vi "acquire-sequence-to-disk-subvi.vi"(0 "Image Size":T4={"H Bin"=1.0, "V Bin"=1.0, "Left"=1.0, "Right"=1024.0, "Top"=1.0, "Bottom"=1024.0} {"V Bin" min=0.0; "H Bin" min=0.0 step=1.0}, 1 "Description Info":string, 2 "Operation":enum16{"Start", "Continue", "Finish"}(ring), 3 "Number of frames to acquire":i32, 5 "Display?":bool, 7 "State In":T1 {"Height" format="%.2f"; "Width" format="%.2f"}, 9 "Frames per acquisition file":u32, 11 "Sequence files handle":T5, 12 "Pressing stop \nautomatically runs finish?":bool=TRUE, 13 "Display Window Title":string="Acquired Image", 14 "Display Window Number":i32) -> (4 "Done?":bool, 6 "State Out":T1 {"Height" format="%.2f"; "Width" format="%.2f"}, 10 "Sequence files handle out":T5, 15 "Error Out":errorcluster)   [LabVIEW 2014]
uses:
  ctt's/Video acquisition state1.ctl
  <vilib>/vision/Image Controls.llb/IMAQ Image.ctl
  ctt's/Header2 file.ctl
  Globals/Initilize Globals.vi
  Stage Control/stage-controller-globals.vi
  Shutter Control/Shutter SubVIs/Global Shutter Variables - SubVI.vi
  Globals/flow-rate-global.vi
  Globals/Andor Camera Temperature.vi
  Globals/hardware names - global.vi
panel:
  in  "Laser Shutter (to get strings only)":T3(radio)
  out "Frame interval (ms)":i16
  out "TTB element zero":u32
  out "Time of 1st frame":dbl
  out "Frames Acquired":u32(slide) scale=0.0..10000.0
  in  "Stop":bool
  out "Sequence files directory path":path
  # "Outputs"
  # "Inputs"
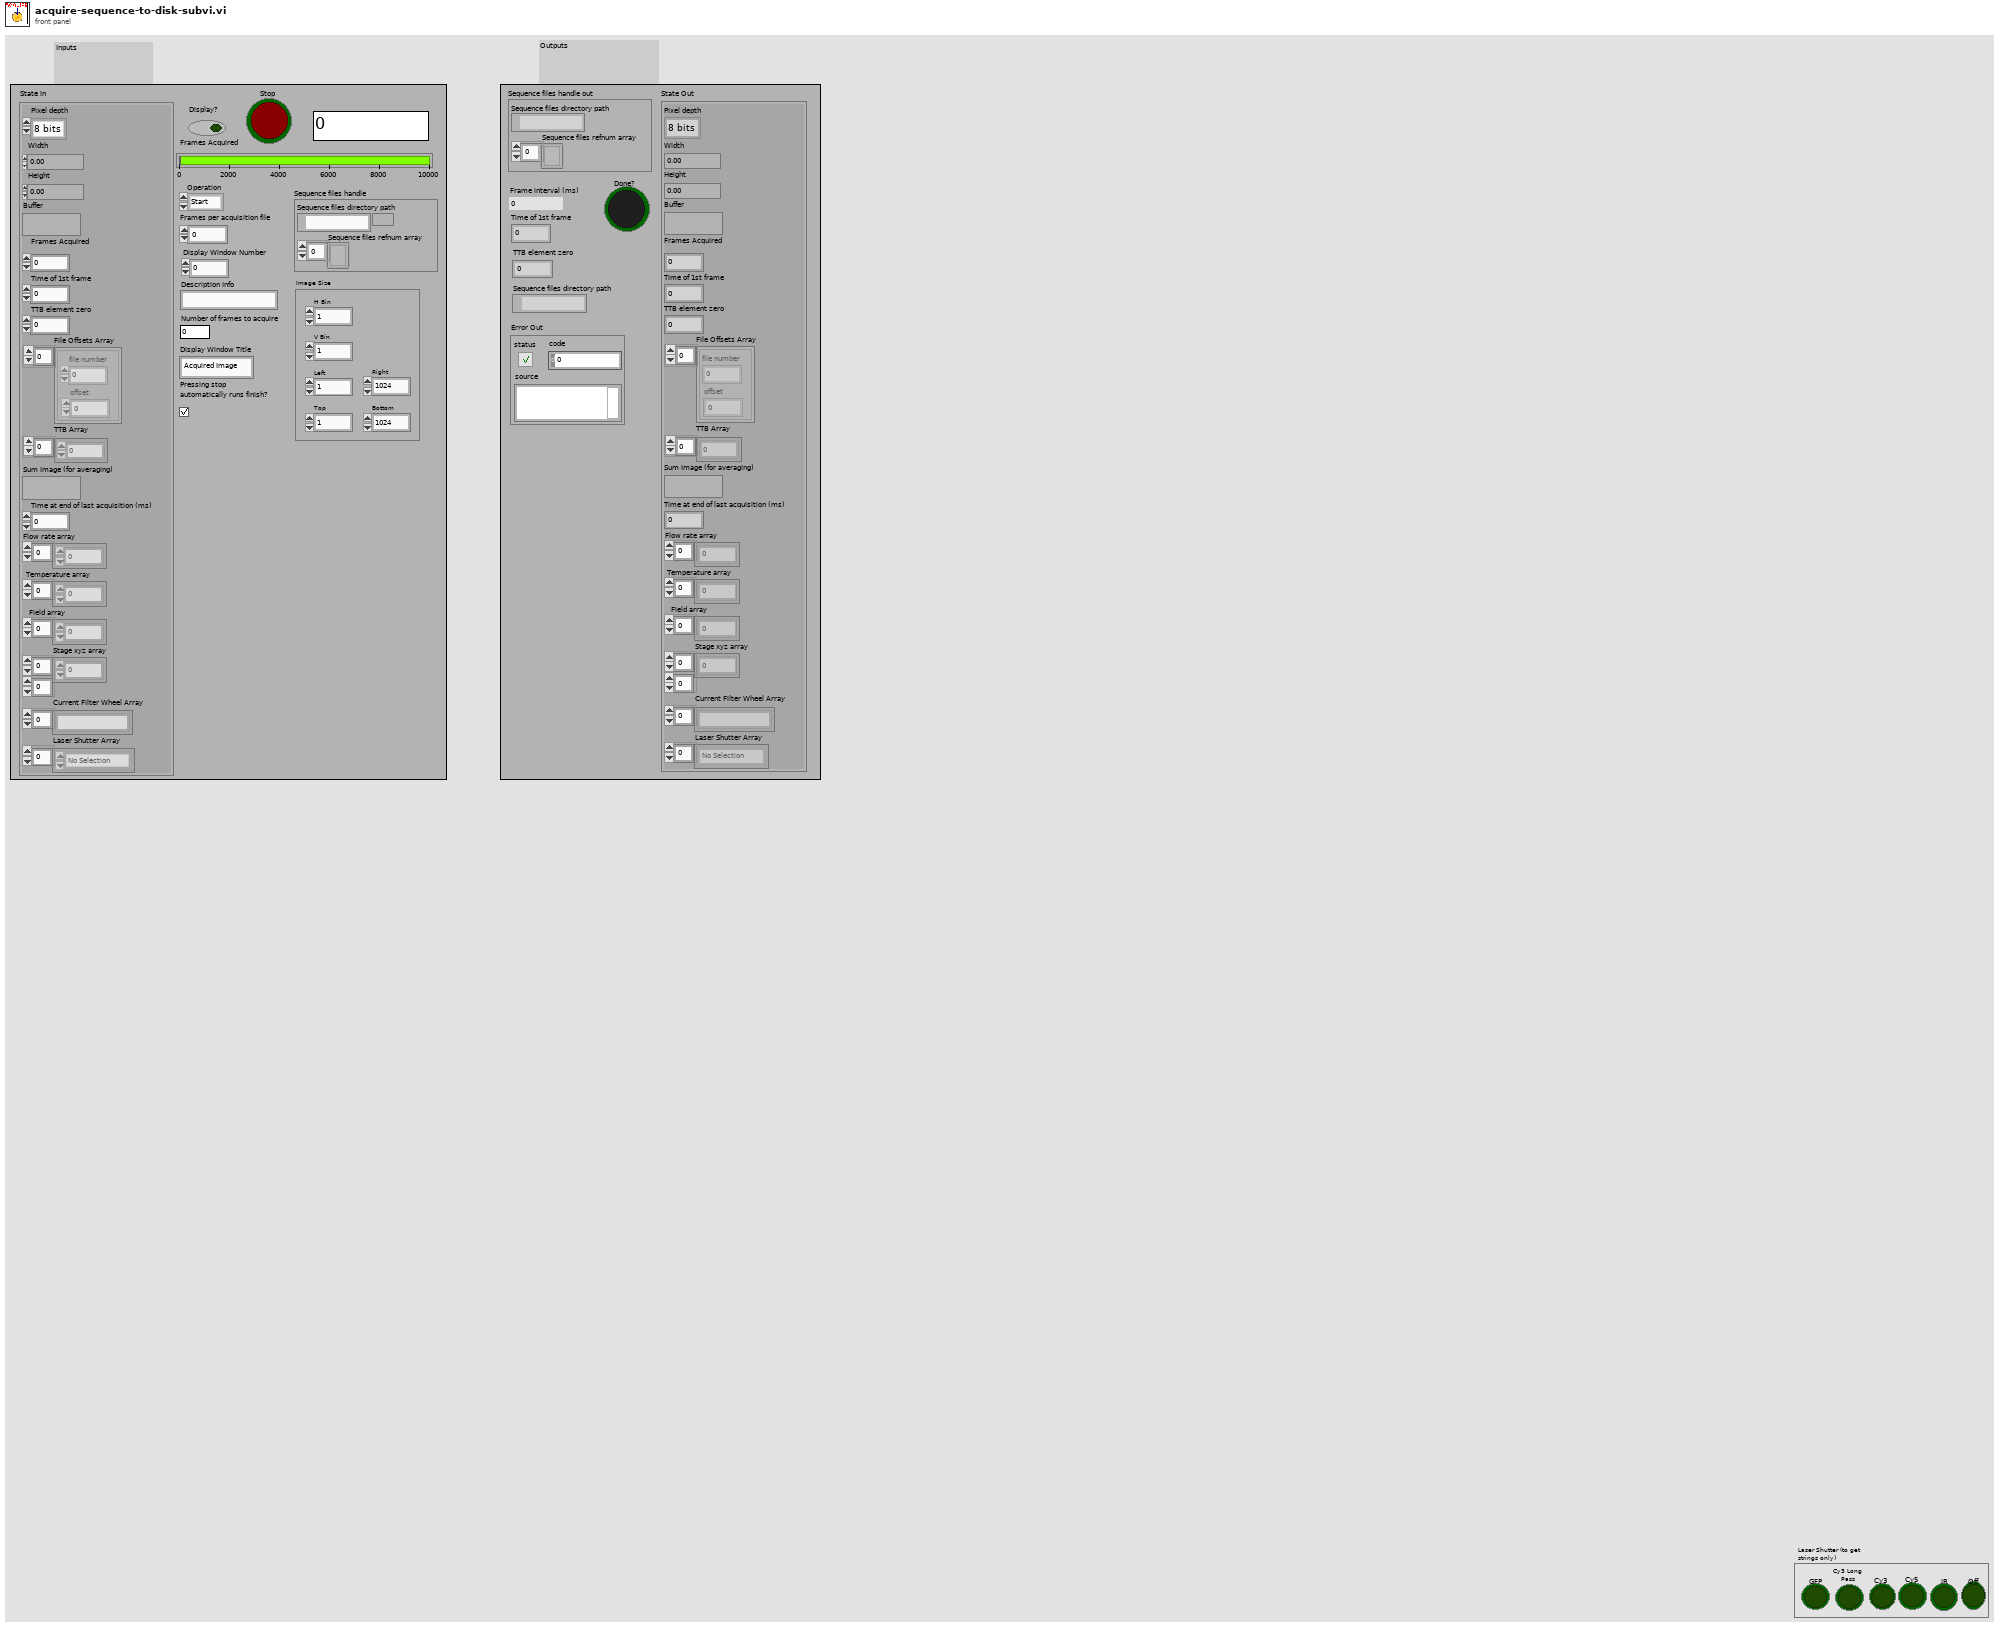
[diagram p1: front panel]
types:
  T1 = typedef "Video acquisition state1.ctl" = cluster{"Pixel depth":enum32{"8 bits", "16 bits", "Float", "Complex", "RGB Chunky", "Compressed"}, "Width":dbl, "Height":dbl, "Buffer":T2, "Frames Acquired":u32, "Time of 1st frame":dbl, "TTB element zero":u32, "File Offsets Array":cluster{"offset":i32, "file number":u8}[], "TTB Array":u32[], "Sum Image (for averaging)":T2, "Time at end of last acquisition (ms)":u32, "Flow rate array":dbl[], "Temperature array":dbl[], "Field array":u16[], "Stage xyz array":dbl[][], "Current Filter Wheel Array":string[], "Laser Shutter Array":enum32{"No Selection", "GFP", "Cy3 Long \nPass", "Cy3", "Cy5", "Off", "IR"}[]}
  T2 = typedef "IMAQ Image.ctl" = refnum<image>
  T3 = enum32{"No Selection", "GFP", "Cy3 Long \nPass", "Cy3", "Cy5", "Off", "IR"}
  T4 = cluster{"H Bin":dbl, "V Bin":dbl, "Left":dbl, "Right":dbl, "Top":dbl, "Bottom":dbl}
  T5 = cluster{"Sequence files directory path":path, "Sequence files refnum array":refnum<file>[]}
  T6 = enum32{"8 bits", "16 bits", "Float", "Complex", "RGB Chunky", "Compressed"}
  T7 = enum32{"No Selection", "GFP", "Cy3 Long \nPass", "Cy3", "Cy5", "Off", "IR"}[]
  T8 = typedef "laser shutters.ctl" = enum32{"No Selection", "GFP", "Cy3 Long \nPass", "Cy3", "Cy5", "Off", "IR"}
  T9 = typedef "Header2 file.ctl" = cluster{"Camera":string, "Microscope":string, "Microscope software version":string, "Flow rate array":dbl[], "Temperature array":dbl[], "Field array":u16[], "Is header2 info present?":bool, "Description Info":string, "Stage xyz array":dbl[][], "Current Filter Wheel Array":string[], "Laser Shutter Array":enum32{"No Selection", "GFP", "Cy3 Long \nPass", "Cy3", "Cy5", "Off", "IR"}[], "Laser Shutter Names":string[]}
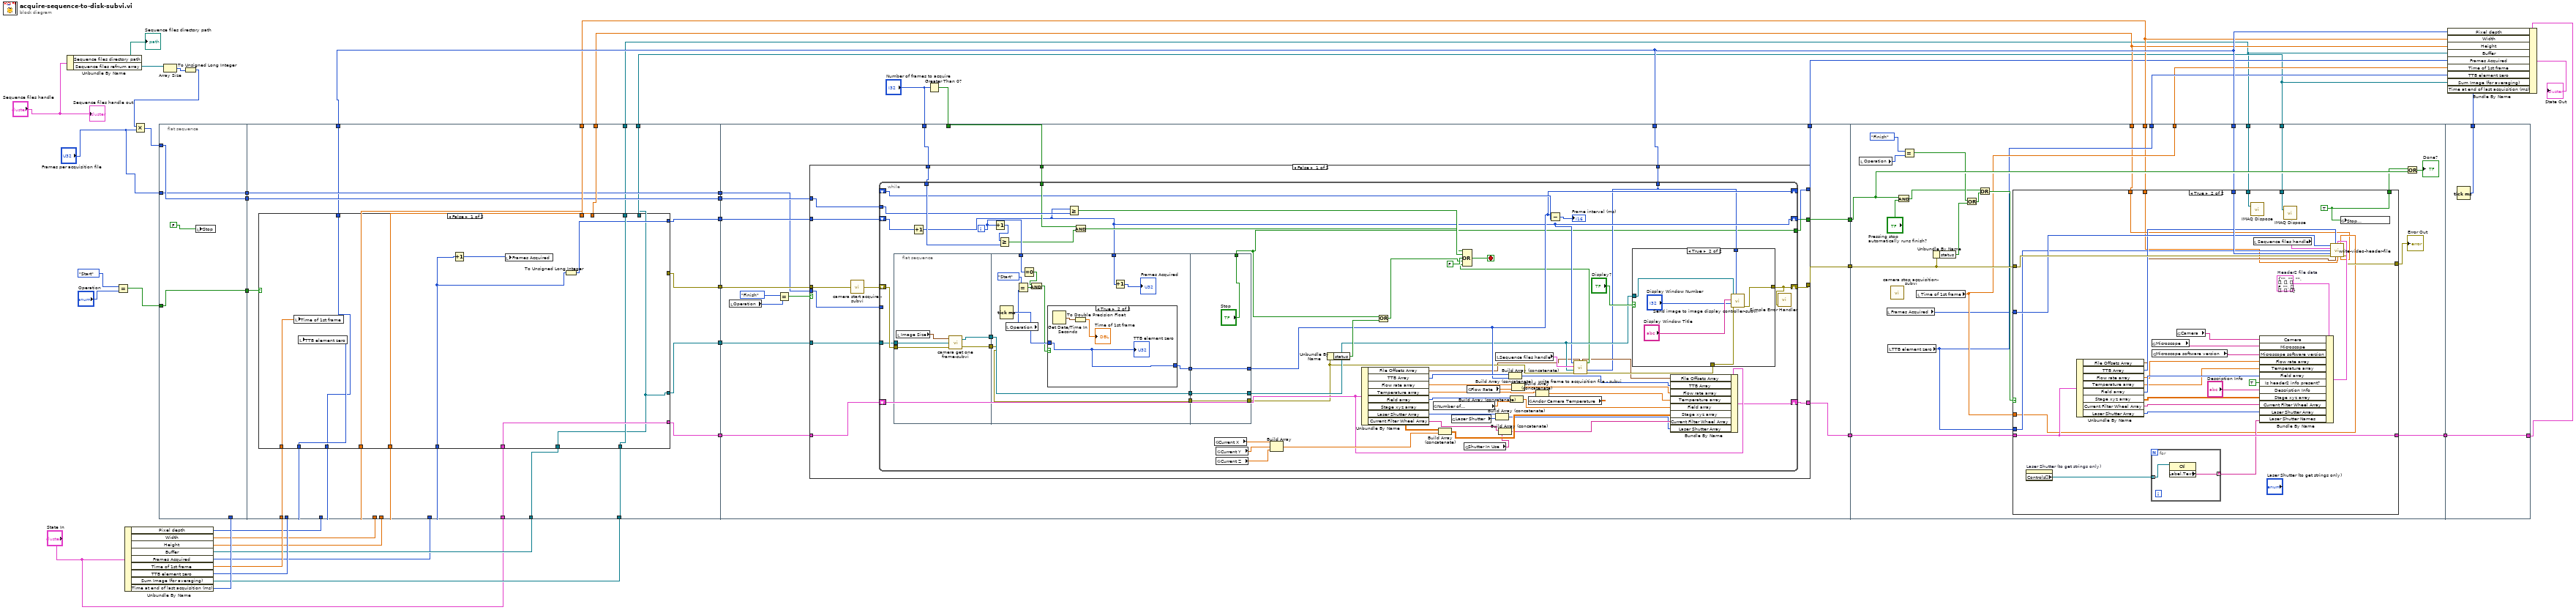
[diagram p0: block diagram]
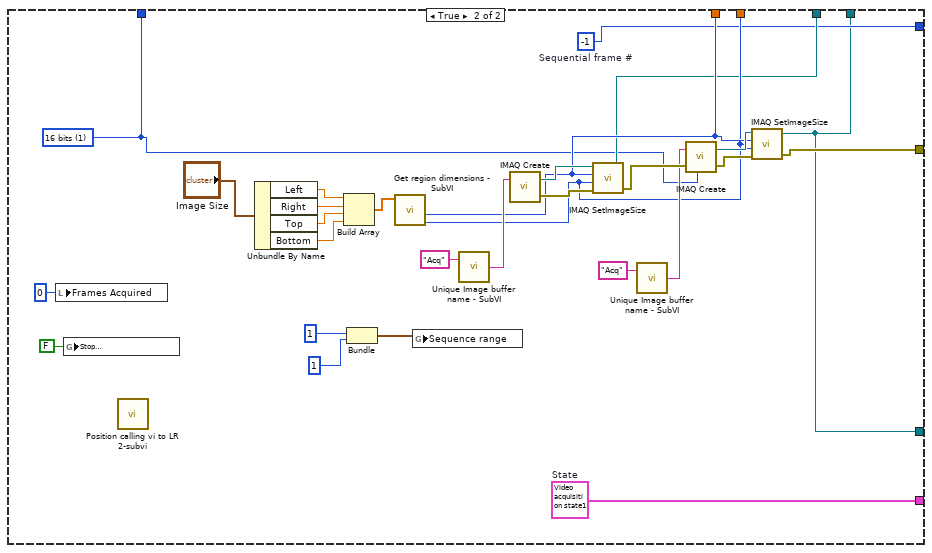
[diagram p2: hidden frame]
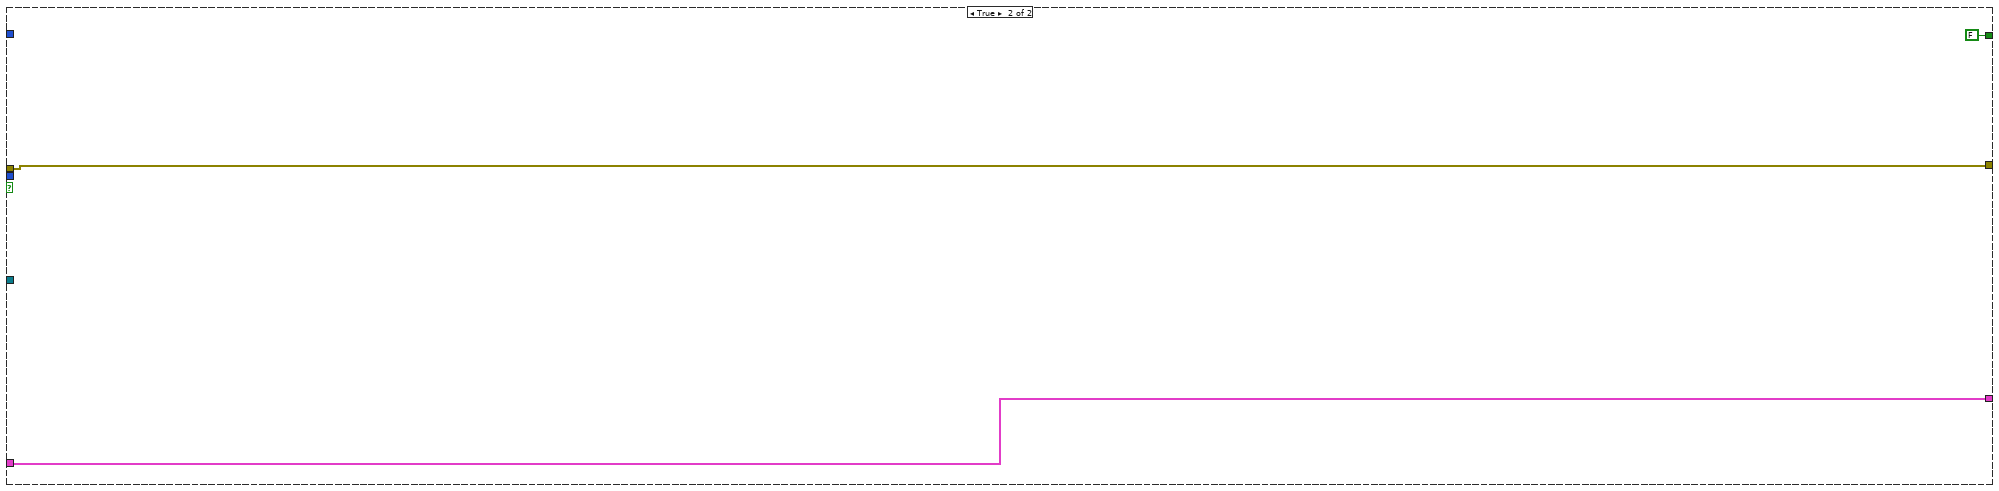
[diagram p5: hidden frame]
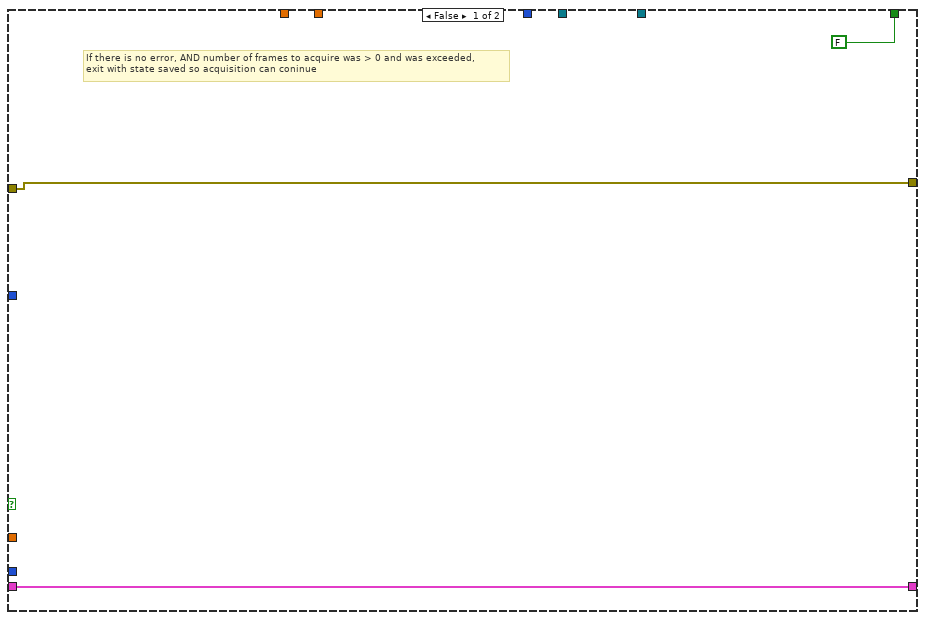
[diagram p6: hidden frame]
diagram:
  n1 = Unbundle By Name("Sequence files handle") -> ("Sequence files directory path"=→"Sequence files directory path":path, "Sequence files refnum array"=w44:refnum<file>[])
  n2 = Equal?(x=enum16{"Start", "Continue", "Finish"}."Start" ("Operation"), y="Operation") -> (x = y?=w38:bool)
  n3 = Unbundle By Name("State In") -> ("Pixel depth"=w29:T6, "Width"=w32:dbl, "Height"=w31:dbl, "Buffer"=w30:T2, "Frames Acquired"=w28:u32, "Time of 1st frame"=w34:dbl, "TTB element zero"=w33:u32, "Sum Image (for averaging)"=w35:T2, "Time at end of last acquisition (ms)"=w36:u32)
  n4 = flat-sequence {
    tunnel: w42 -> [w48]
    tunnel: w38 -> [w50]
    tunnel: [w50] -> w37
    tunnel: w36 -> [_]
    tunnel: [w48] -> w24
    tunnel: "Frames per acquisition file" -> [w47]
    tunnel: [w47] -> w21
    tunnel: w37 -> [w71]
    tunnel: w35 -> [w62]
    tunnel: w34 -> [w70]
    tunnel: w33 -> [w69]
    tunnel: w32 -> [w67]
    tunnel: w31 -> [w66]
    tunnel: "State In" -> [w64]
    tunnel: w30 -> [w63]
    tunnel: w29 -> [w68]
    tunnel: w28 -> [w65]
    tunnel: [w61] -> w7
    tunnel: [w60] -> w6
    tunnel: [w59] -> w27
    tunnel: [w58] -> w26
    tunnel: [w57] -> w25
    tunnel: w24 -> [w57]
    tunnel: [w56] -> w22
    tunnel: w21 -> [w56]
    tunnel: [w55] -> w20
    tunnel: [w54] -> w17
    tunnel: [w53] -> w8
    tunnel: [w52] -> w1
    tunnel: [w51] -> w2
    tunnel: w27 -> [w123]
    tunnel: w26 -> [w122]
    tunnel: w25 -> [w121]
    tunnel: w22 -> [w120]
    tunnel: w20 -> [w119]
    tunnel: w19 -> [w117]
    tunnel: "Number of frames to acquire" -> [w118]
    tunnel: w17 -> [w116]
    tunnel: w8 -> [w115]
    tunnel: [w112] -> w16
    tunnel: [w114] -> w15
    tunnel: [w113] -> w14
    tunnel: [w111] -> w3
    tunnel: w16 -> [w245]
    tunnel: w15 -> [w255]
    tunnel: w14 -> [w254]
    tunnel: [w248] -> w4
    tunnel: [w247] -> w5
    tunnel: w1 -> [w241]
    tunnel: w2 -> [w240]
    tunnel: w6 -> [w239]
    tunnel: w7 -> [w238]
    tunnel: w8 -> [w237]
    tunnel: [w236] -> w12
    tunnel: w12 -> [w295]
    tunnel: [w295] -> w11
    tunnel: [w294] -> w9
    frame #0 {
      n5 = local write "Stop"(FALSE) -> ()
    }
    frame #1 {
      n6 = case shown="False" w71 {
        tunnel: w70 -> [w80 _]
        tunnel: w69 -> [w79 _]
        tunnel: w68 -> [w78 _]
        tunnel: w67 -> [w74 _]
        tunnel: w66 -> [w73 _]
        tunnel: w65 -> [w76 _]
        tunnel: w64 -> [w82 _]
        tunnel: w63 -> [w72 _]
        tunnel: w62 -> [w81 _]
        tunnel: [w78 w85] -> w53
        tunnel: [w82 w95] -> w54
        tunnel: [w74 w89] -> w61
        tunnel: [w73 w88] -> w60
        tunnel: [_ w87] -> w59
        tunnel: [w72 w83] -> w51
        tunnel: [w81 w86] -> w52
        tunnel: [w75 w84] -> w58
        tunnel: [w72 w83] -> w55
        frame False {
          n7 = local write "Time of 1st frame"(w80) -> ()
          n8 = local write "TTB element zero"(w79) -> ()
          n9 = Increment(x=w76) -> (x+1=w77:u32)
          n10 = local write "Frames Acquired"(w77) -> ()
          n11 = To Unsigned Long Integer(number=w76) -> (unsigned 32bit integer=w75:u32)
        }
        frame True {
          w84 = -1  # Sequential frame #
          w85 = u32 1 items=["8 bits", "16 bits", "Float", "Complex", "RGB", "HSL"] ("Image Type")
          w95 = T1 {"Pixel depth"=enum."8 bits", "Width"=0.0, "Height"=0.0, "Buffer"=refnum, "Frames Acquired"=0, "Time of 1st frame"=0.0, "TTB element zero"=0, "File Offsets Array"=[], "TTB Array"=[], "Sum Image (for averaging)"=refnum, "Time at end of last acquisition (ms)"=0, "Flow rate array"=[], "Temperature array"=[], "Field array"=[], "Stage xyz array"=[], "Current Filter Wheel Array"=[], "Laser Shutter Array"=[]}  # State
          n12 = local write "Frames Acquired"(u32 0 ("Frames Acquired")) -> ()
          n13 = global write "Initilize Globals.vi" "Stop \nAcquisition"(FALSE ("Stop \nAcquisition")) -> ()
          n14 = call "Position calling vi to LR 2-subvi.vi"() -> ()  [unwired: 4 in, 2 out]
          n15 = Unbundle By Name("Image Size") -> ("Left"=w109:dbl, "Right"=w108:dbl, "Top"=w107:dbl, "Bottom"=w106:dbl)
          n16 = Build Array(w109, w108, w107, w106) -> (w100:dbl[])
          n17 = Bundle(1, 1) -> (w101:cluster{i32, i32})  [unwired: 1 in]
          n18 = call "Get region dimensions - SubVI.vi"("x1y1x2y2"=w100) -> ("y size"=w88:u16, "x size"=w89:u16)  [unwired: 7 in, 2 out]
          n19 = global write "Initilize Globals.vi" "Sequence range"(w101) -> ()
          n20 = call "Unique Image buffer name - SubVI.vi"("Buffer  base name"="Acq") -> ("Image Name"=w99:string)  [unwired: 1 in]
          n21 = call "IMAQ Create"("Image Name"=w99) -> ("New Image"=w97:T2, "error out"=w96:errorcluster)  [unwired: 4 in]
          n22 = call "IMAQ SetImageSize"("error in (no error)"=w96, "Y Resolution"=w88, "X Resolution"=w89, "Image"=w97) -> ("error out"=w94:errorcluster, "Image Out"=w86:T2)  [unwired: 1 in]
          n23 = call "Unique Image buffer name - SubVI.vi"("Buffer  base name"="Acq") -> ("Image Name"=w92:string)  [unwired: 1 in]
          n24 = call "IMAQ Create"("Image Name"=w92, "Image Type"=w85, "error in (no error)"=w94) -> ("New Image"=w90:T2, "error out"=w91:errorcluster)  [unwired: 2 in]
          n25 = call "IMAQ SetImageSize"("error in (no error)"=w91, "Y Resolution"=w88, "X Resolution"=w89, "Image"=w90) -> ("error out"=w87:errorcluster, "Image Out"=w83:T2)  [unwired: 1 in]
        }
      }
    }
    frame #2 {
      n26 = local read "Operation"() -> (w125:enum16{"Start", "Continue", "Finish"})
      n27 = Equal?(x=enum16{"Start", "Continue", "Finish"}."Finish" ("Operation"), y=w125) -> (x = y?=w124:bool)
      n28 = case shown="False" w124 {
        tunnel: w123 -> [w140 w235]
        tunnel: w122 -> [w138 _]
        tunnel: w121 -> [w137 _]
        tunnel: w120 -> [w136 _]
        tunnel: w119 -> [w135 _]
        tunnel: w118 -> [w134 _]
        tunnel: w117 -> [w133 _]
        tunnel: w116 -> [w132 w233]
        tunnel: [w131 w235] -> w113
        tunnel: w115 -> [w130 _]
        tunnel: [w129 w233] -> w112
        tunnel: [w128 FALSE ("Stop")] -> w114
        tunnel: [w127 _] -> w111
        frame False {
          n29 = call "camera start acquire - subvi.vi"("error in"=w140) -> ("error out"=w139:errorcluster)
          n30 = while {
            shift-right: [w172] -> w131
            shift-left: w139 -> [w200]
            shift-right: [w151] -> w127
            shift-left: w138 -> [w190]
            tunnel: w137 -> [w189]
            tunnel: w136 -> [_]
            tunnel: w135 -> [w199]
            tunnel: w134 -> [w191]
            tunnel: w133 -> [w187]
            shift-right: [w165] -> w129
            shift-left: w132 -> [w166]
            shift-right: [w156] -> _
            shift-left: _ -> [w175]
            tunnel: w130 -> [w146]
            tunnel: [w145] -> w128
            i -> [w193]
            stop <- w186 stop-if-true
            n31 = flat-sequence {
              tunnel: w200 -> [w211]
              tunnel: w199 -> [w210]
              tunnel: [w209] -> w198
              tunnel: [w208] -> w197
              tunnel: w198 -> [w216]
              tunnel: w197 -> [w217]
              tunnel: [w217] -> w196
              tunnel: [w216] -> w195
              tunnel: [w215] -> w194
              tunnel: w193 -> [w214]
              tunnel: w151 -> [w213]
              tunnel: [w231] -> w152
              tunnel: [w232] -> w153
              tunnel: w196 -> [w232]
              tunnel: w195 -> [w231]
              tunnel: [w230] -> w156
              tunnel: w194 -> [w230]
              tunnel: ["Stop"] -> w145
              frame #0 {
                n32 = local read "Image Size"() -> (w212:T4)
                n33 = call "camera get one frame-subvi.vi"("error in"=w211, "New Image"=w210, "Image Size"=w212) -> ("error out"=w209:errorcluster, "Image Out"=w208:T2)
              }
              frame #1 {
                n34 = Tick Count (ms)() -> (millisecond timer value=w224:u32)
                n35 = local read "Operation"() -> (w219:enum16{"Start", "Continue", "Finish"})
                n36 = Equal?(x=enum16{"Start", "Continue", "Finish"}."Start" ("Operation"), y=w219) -> (x = y?=w221:bool)
                n37 = Equal To 0?(x=w214) -> (x = 0?=w218:bool)
                n38 = And(x=w218, y=w221) -> (x .and. y?=w222:bool)
                n39 = case shown="True" w222 {
                  tunnel: w224 -> [w225 w228]
                  tunnel: [w225 w228] -> w215
                  frame False {
                  }
                  frame True {
                    n40 = Get Date/Time In Seconds() -> (seconds since 1Jan1904=w227:timestamp)
                    n41 = To Double Precision Float(number=w227) -> (double precision float=→"Time of 1st frame":dbl)
                    "TTB element zero" <- w228
                  }
                }
                n42 = Increment(x=w213) -> (x+1=→"Frames Acquired":u32)
              }
              frame #2 {
              }
            }
            n43 = Increment(x=w190) -> (x+1=w151:u32)
            n44 = Increment(x=w193) -> (x+1=w192:i32)
            n45 = Greater Or Equal?(x=w192, y=w191) -> (x >= y?=w188:bool)
            n46 = Greater Or Equal?(x=w151, y=w189) -> (x >= y?=w184:bool)
            n47 = And(x=w187, y=w188) -> (x .and. y?=w183:bool)
            n48 = global read "stage-controller-globals.vi" "Current X"() -> (w180:dbl)
            n49 = global read "stage-controller-globals.vi" "Current Y"() -> (w179:dbl)
            n50 = global read "stage-controller-globals.vi" "Current Z"() -> (w178:dbl)
            n51 = Build Array(w180, w179, w178) -> (w177:dbl[])
            n52 = Unbundle By Name(w152) -> ("status"=w181:bool)
            n53 = Unbundle By Name(w166) -> ("File Offsets Array"=w148:cluster{"offset":i32, "file number":u8}[], "TTB Array"=w171:u32[], "Flow rate array"=w169:dbl[], "Temperature array"=w143:dbl[], "Field array"=w170:u16[], "Stage xyz array"=w176:dbl[][], "Laser Shutter Array"=w168:T7, "Current Filter Wheel Array"=w167:string[])
            n54 = Or(x=w145, y=w181) -> (x .or. y?=w182:bool)
            n55 = global read "stage-controller-globals.vi" "Number of \nField Steps"() -> (w144:dbl)
            n56 = Build Array (concatenate)(w176, w177) -> (w164:dbl[][])
            n57 = global read "Global Shutter Variables - SubVI.vi" "Laser Shutter"() -> (w161:T8)
            n58 = global read "Global Shutter Variables - SubVI.vi" "Shutter In Use"() -> (w163:string)
            n59 = global read "flow-rate-global.vi" "Flow Rate"() -> (w158:dbl)
            n60 = local read "Sequence files handle"() -> (w154:T5)
            n61 = Build Array (concatenate)(w168, w161) -> (w160:T8[])
            n62 = Build Array (concatenate)(w167, w163) -> (w162:string[])
            n63 = Build Array (concatenate)(w171, w156) -> (w155:u32[])
            n64 = Build Array (concatenate)(w170, w144) -> (w159:dbl[])
            n65 = Build Array (concatenate)(w169, w158) -> (w157:dbl[])
            n66 = global read "Andor Camera Temperature.vi" "Andor Camera Temperature"() -> (w141:dbl)
            n67 = Build Array (concatenate)(w143, w141) -> (w142:dbl[])
            n68 = Subtract(x=w156, y=w175) -> (x-y=→"Frame interval (ms)":u32)
            n69 = call "write frame to acquisition file - subvi.vi"("Pixel depth"=w146, "Offset table in"=w148, "Error In"=w152, "Image In"=w153, "Sequence files handle"=w154, "Last frame number written in"=w151) -> ("Error Out"=w149:errorcluster, "Stop"=w150:bool, "Offset table out"=w147:cluster{"offset":i32, "file number":u8}[])  [unwired: 2 in, 1 out]
            n70 = Compound Arithmetic op=OR(w183, w184, FALSE, w182, w150) -> (w186:bool)
            n71 = case shown="True" "Display?" {
              tunnel: [w201 w207] -> w172
              tunnel: w149 -> [w201 w204]
              tunnel: w153 -> [_ w203]
              tunnel: w146 -> [_ w202]
              frame False {
              }
              frame True {
                n72 = call "Send image to image display controller-subvi.vi"("Image"=w203, "Window Title"="Display Window Title", "Window Number"="Display Window Number", "error in"=w204, "Image Type"=w202) -> ("error out"=w207:errorcluster)  [unwired: 4 in, 1 out]
              }
            }
            n73 = Bundle By Name(cluster=w166, "File Offsets Array"=w147, "TTB Array"=w155, "Flow rate array"=w157, "Temperature array"=w142, "Field array"=w159, "Stage xyz array"=w164, "Current Filter Wheel Array"=w162, "Laser Shutter Array"=w160) -> (w165:T1)
            n74 = call <vilib>:"Simple Error Handler.vi"("error in (no error)"=w172) -> ()  [unwired: 4 in, 5 out]
          }
        }
        frame True {
        }
      }
    }
    frame #3 {
      n75 = local read "Operation"() -> (w258:enum16{"Start", "Continue", "Finish"})
      n76 = local read "Frames Acquired"() -> (w246:u32)
      n77 = local read "TTB element zero"() -> (w247:u32)
      n78 = call "camera stop acquisition- subvi.vi"() -> ()  [unwired: 1 in]
      n79 = And(x=w255, y="Pressing stop \nautomatically runs finish?") -> (x .and. y?=w251:bool)
      n80 = Equal?(x=enum16{"Start", "Continue", "Finish"}."Finish" ("Operation"), y=w258) -> (x = y?=w252:bool)
      n81 = local read "Time of 1st frame"() -> (w248:dbl)
      n82 = Unbundle By Name(w254) -> ("status"=w253:bool)
      n83 = Or(x=w252, y=w253) -> (x .or. y?=w250:bool)
      n84 = Or(x=w251, y=w250) -> (x .or. y?=w249:bool)
      n85 = case shown="True" w249 {
        tunnel: w254 -> [w260 w272]
        tunnel: w248 -> [_ w265]
        tunnel: w247 -> [_ w266]
        tunnel: w246 -> [_ w269]
        tunnel: w245 -> [w261 w291]
        tunnel: [w261 w291] -> w236
        tunnel: [w260 w273] -> w244
        tunnel: [FALSE w262] -> w243
        tunnel: w241 -> [_ w278]
        tunnel: w240 -> [_ w277]
        tunnel: w239 -> [_ w264]
        tunnel: w238 -> [_ w263]
        tunnel: w237 -> [_ w271]
        frame False {
          # "If there is no error, AND number of frames to acquire was > 0 and was exceeded,\nexit with state saved so acquisition can coninue"
        }
        frame True {
          w290 = T9 {"Camera"="", "Microscope"="", "Microscope software version"="", "Flow rate array"=[], "Temperature array"=[], "Field array"=[], "Is header2 info present?"=FALSE, "Description Info"="", "Stage xyz array"=[], "Current Filter Wheel Array"=[], "Laser Shutter Array"=[], "Laser Shutter Names"=[]}  # Header2 file data
          w262 = TRUE
          n86 = property on="Laser Shutter (to get strings only)" class="RadioBtnsControl (strict)"() -> ("Controls[]"=w276:refnum<vi>[])  [unwired: 2 in, 2 out]
          n87 = Unbundle By Name(w291) -> ("File Offsets Array"=w267:cluster{"offset":i32, "file number":u8}[], "TTB Array"=w268:u32[], "Flow rate array"=w284:dbl[], "Temperature array"=w285:dbl[], "Field array"=w289:u16[], "Stage xyz array"=w286:dbl[][], "Current Filter Wheel Array"=w287:string[], "Laser Shutter Array"=w288:T7)
          n88 = for {
            tunnel: w276 -> [w293] mode=indexing
            tunnel: [w292] -> w275 mode=indexing
            n89 = property class="Ctl"(reference=w293) -> ("Label.Text"=w292:string)  [unwired: 1 in, 2 out]
          }
          n90 = global read "hardware names - global.vi" "Microscope"() -> (w280:string)
          n91 = global read "hardware names - global.vi" "Microscope software version"() -> (w279:string)
          n92 = global read "hardware names - global.vi" "Camera"() -> (w281:string)
          n93 = call "IMAQ Dispose"("Image"=w278) -> ()  [unwired: 2 in, 4 out]
          n94 = local read "Sequence files handle"() -> (w270:T5)
          n95 = Bundle By Name(cluster=w290, "Camera"=w281, "Microscope"=w280, "Microscope software version"=w279, "Flow rate array"=w284, "Temperature array"=w285, "Field array"=w289, "Is header2 info present?"=TRUE, "Description Info"="Description Info", "Stage xyz array"=w286, "Current Filter Wheel Array"=w287, "Laser Shutter Array"=w288, "Laser Shutter Names"=w275) -> (w274:T9)
          n96 = call "IMAQ Dispose"("Image"=w277) -> ()  [unwired: 2 in, 4 out]
          n97 = call "write-video-header-file.vi"("Frames Acquired"=w269, "TTB Array (ms)"=w268, "Header2 file data"=w274, "time of 1st frame, \nsec"=w265, "Sequence files handle"=w270, "Element 0 of TTB"=w266, "Pixel depth\n(0=8 bit; 1= 16 bit)"=w271, "Error In"=w272, "File Offsets Array"=w267, "Region width"=w263, "Region height"=w264) -> ("Error Out"=w273:errorcluster)  [unwired: 4 in]
          n98 = global write "Initilize Globals.vi" "Stop \nAcquisition"(w262) -> ()
        }
      }
      "Error Out" <- w244
      n99 = Or(x=w243, y=w255) -> (x .or. y?=→"Done?":bool)
    }
    frame #4 {
      n100 = Tick Count (ms)() -> (millisecond timer value=w294:u32)
    }
  }
  n101 = Array Size(array=w44) -> (size(s)=w43:i32)
  n102 = To Unsigned Long Integer(number=w43) -> (unsigned 32bit integer=w41:u32)
  n103 = Multiply(x=w41, y="Frames per acquisition file") -> (x*y=w42:u32)
  n104 = Greater Than 0?(x="Number of frames to acquire") -> (x > 0?=w19:bool)
  n105 = Bundle By Name(cluster=w11, "Pixel depth"=w8, "Width"=w7, "Height"=w6, "Buffer"=w1, "Frames Acquired"=w3, "Time of 1st frame"=w4, "TTB element zero"=w5, "Sum Image (for averaging)"=w2, "Time at end of last acquisition (ms)"=w9) -> (→"State Out":T1)
  "Sequence files handle out" <- "Sequence files handle"
